vi "Parse State Queue++.vi"(0 "State Queue":string, 1 "Name(\"\" to use uuid)":string, 2 "Response Arguments":string, 7 "Error In (no error)":errorcluster, 9 "Dequeue Timeout(0ms)":i32, 11 "Response Timeout(5000ms)":i32=5000, 12 "Allowed Messages(Empty for all)":string[](array[string])) -> (3 "Name Used":string, 4 "Remaining States":string, 6 "Current State":string, 8 "Arguments":string, 10 ">> Response Source Message >>":T1, 15 ">> Source CSM >>":string)   [LabVIEW 2020, in "Communicable State Machine.lvlib"]
doc: "Parses the CSM state queue and returns the current state that will execute next with the associated arguments.\n\n\n<b>Inputs:</b>\n - <b>State Queue</b>: The entire state queue is wired to this input. This should come from the main CSM shift register.\n - <b>Error In (no error)</b>: The error cluster from the CSM is wired to this input. If an error occures and appears on this input, the current state output returns the \"Error Handler\" state.\n - <b>Name(\"\" to use uuid)</b>: Module Name\n - If Input is \"\", an uuid will be used for module name. The module is marked as stand-alone mode and will not be included in module list.\n - Fi Input end with '#', the module will worked in worker mode. Modules with the same name will shared the same message queue. Any external message will be processed by one of the modules, depends on who is free.\n - Otherwise, the input string will be used as module name, which should be unique in system. CSM will go to \"Critical Error\" state if duplicated module name is used in system.\n - <b>Response Timeout(5000ms)</b>: The timeout of waiting for response of sync-call from outside.\n - <b>Dequeue Timeout(0ms)</b>: The timeout of checking CSM message queue.\n - <b>Response Arguments</b>: The response arguments from last state. It should come from the CSM shift register.\n\n<b>Outputs:</b>\n - <b>Remaining States</b>: Returns all the next states that should execute after the current state completes. These should be passed through the current state in the state machine. These can also be modified or augmented within the current state if necessary.\n - <b>Arguments</b>: Returns any argument(s) that may be used in the current state string. These arguments come after the \">>\" characters. <b>Note:</b> The arguments variable must not contain any unprintable characters like linefeed or carriage return.\n - <b>Current State</b>: The state to be processed\n - <b>Name Used</b>: The actual name assigned to this CSM module\n - <b>Argument - State</b>: If any core error occurs, this is the source state name\n - <b>From Who</b>: If <b>Current State</b> is called by ouside, this is the source CSM module name."
uses:
  Communicable State Machine.lvlib
  _CSM_Response Source Message.ctl
  _CSM_GlobalLog_MSG.ctl
  _CSM_GlobalLog_MSG_TYPE.ctl
  Priority Queue.lvclass/Priority Queue.ctl
  _CSM_MSG_TYPE.ctl
  _CSM Status Change Event Data.ctl
  _CSMObj-Message Check.vi
  _CSMObj-Enqueue Cross-Module Message.vi
  _CSMOFGV Get.vi
  GEvt-Generate with Rule Check.vi
  Cache-Broadcast Registry Search Result.vi
  CSM - Register Status Change.vi
  CSM - Unregister Status Change.vi
  Hex Str to U8 Data.vi
  CSM - Revert Arguments-Safe String.vi
  Add State(s) to Queue__JKI_lib_State_Machine.vi
  Build Internal State String.vi
  Concatenate State with Arguments.vi
  U8 Data to Hex Str.vi
  Dequeue Element.vi
  CSM - Make String Arguments Safe.vi
  Enqueue Element.vi
  Filter Check.vi
  Trim Both Whitespace.vi
  CSM - Keywords.vi
  global-GEvnt Filter Change Flag.vi
  FGV-GEvt Filter Obj.vi
  Group Check - CSM.vi
  Group Check - LogType.vi
  Group Check - State.vi
  CSM Check - LogType.vi
  CSM Check - State.vi
  CSM Check - StateType.vi
  Group Check - StateType.vi
  _CSMOFGV.vi
  CSM Not Allowed Message.vi
  global-CSMQ FGV Change Flag.vi
  global-Broadcast Cache Change Flag.vi
  Broadcast Item Key.vi
  FGV-BroadcastRegistry.vi
  Parse Register Message.vi
  Parse Unregister Message.vi
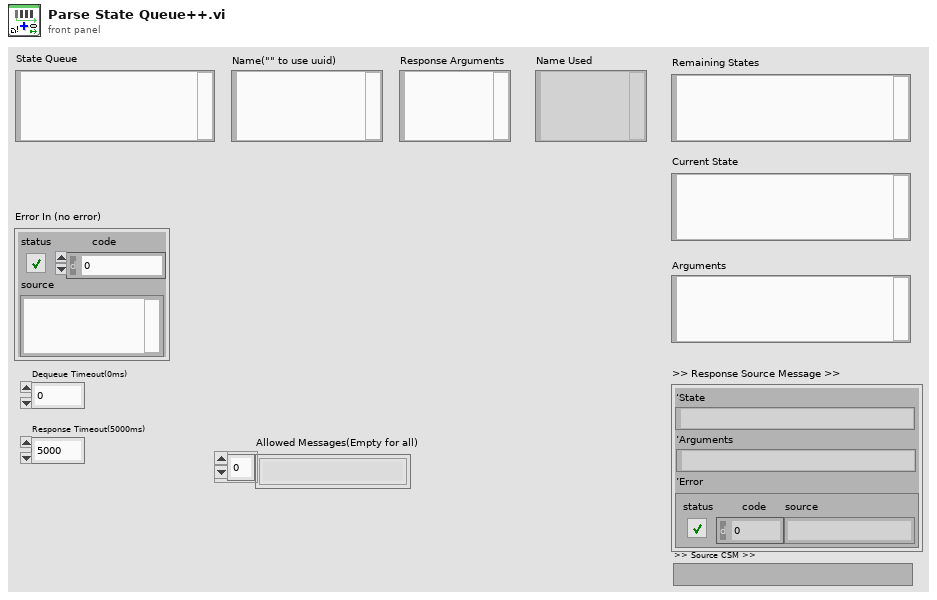
[diagram p1: front panel]
types:
  T1 = typedef "Communicable State Machine.lvlib/_CSM_Response Source Message.ctl" = cluster{"‘State":string, "’Arguments":string, "’Error":errorcluster}
  T2 = typedef "Communicable State Machine.lvlib/_CSM_GlobalLog_MSG.ctl" = cluster{"Name(\"\" to use uuid)":string, "Current State":string, "Arguments":string, "Source Message":T1, "Source Module":string, "Complete(T)/Start(F)":bool, "LogType":T3}
  T3 = typedef "Communicable State Machine.lvlib/_CSM_GlobalLog_MSG_TYPE.ctl" = enum16{"User Log", "State Change", "Status", "Interrupt", "Register", "Unregister", "Error Log", "Module Created", "Module Destroyed"}
  T4 = typedef "Communicable State Machine.lvlib/_CSMObj.ctl" = cluster{"Requested Name":string, "Module Name":string, "Mode":T5, "Queue":refnum<class "Priority Queue.lvclass">, "CSM-Data":refnum<data-value>, "User Event":refnum<user-event>, "Status Change Event":refnum<user-event>, "Allowed Messages":string[], "Mode-Data":refnum<data-value>, "Group Name":string, "Exit Event":refnum<user-event>}
  T5 = typedef "Communicable State Machine.lvlib/_CSM_MODE.ctl" = enum16{"Not Exist", "Stand Alone", "CSM", "Worker Agent", "Worker", "Chain", "Chain Node"}
  T6 = typedef "Communicable State Machine.lvlib/_CSM_MSG_TYPE.ctl" = enum16{"Sync Message(-@)", "Async Message(->)", "Async without Response(->|)", "Async Response", "Broadcast(-><all>)", "Broadcast(-><status>)", "Broadcast(-><interrupt>)", "Append to JKISM States", "Append to JKISM States(High Priority)"}
  T7 = typedef "Communicable State Machine.lvlib/_CSM Status Change Event Data.ctl" = cluster{"ModuleName":string, "Status":string, "Arguments":string}
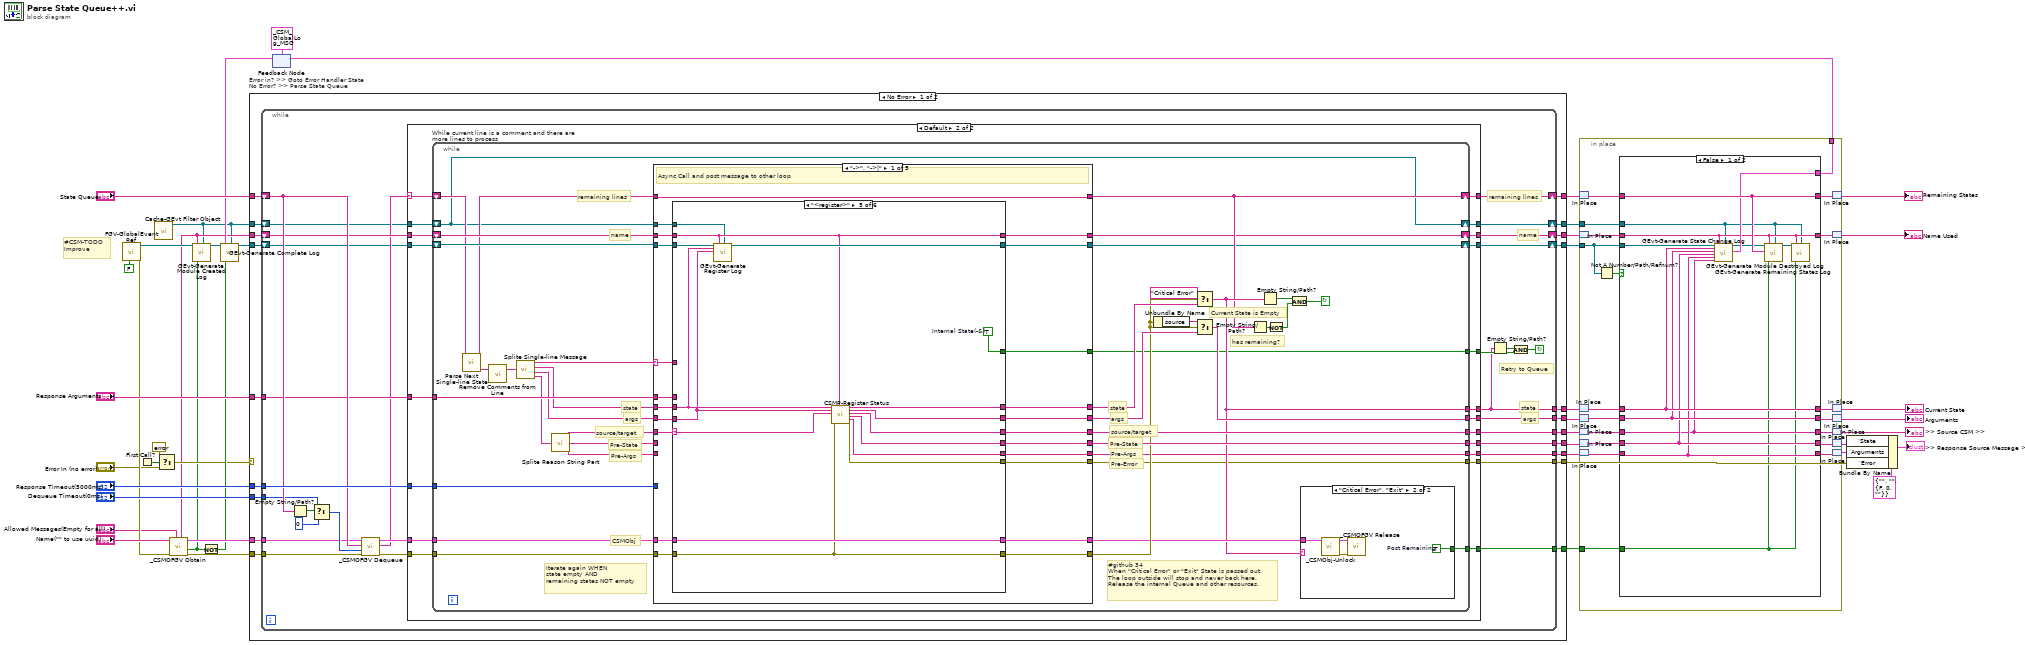
[diagram p0: block diagram]
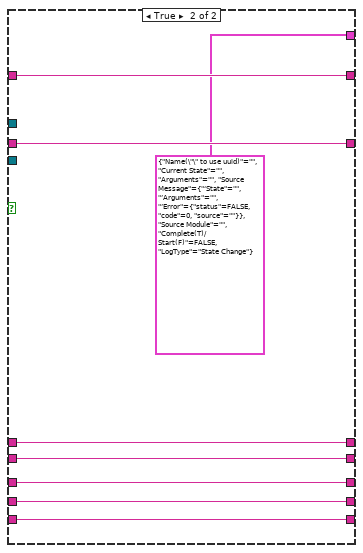
[diagram p2: hidden frame]
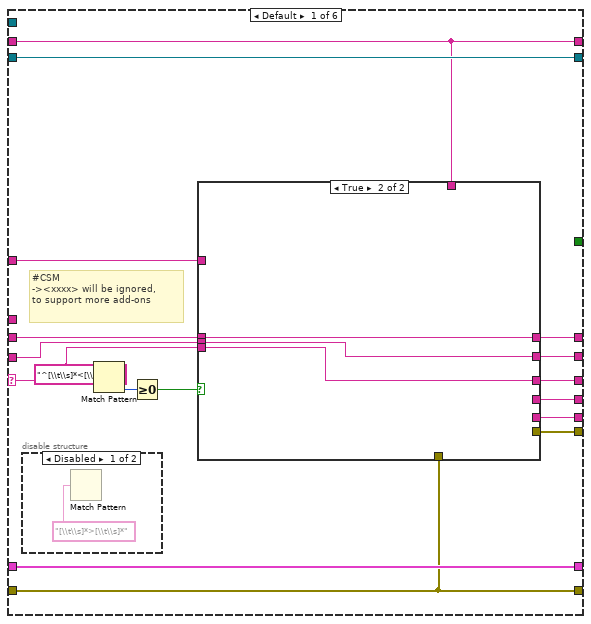
[diagram p5: hidden frame]
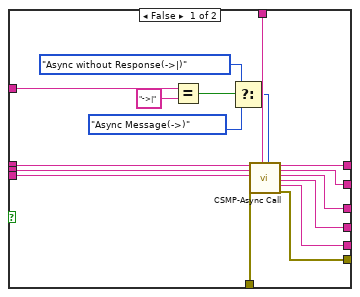
[diagram p7: hidden frame]
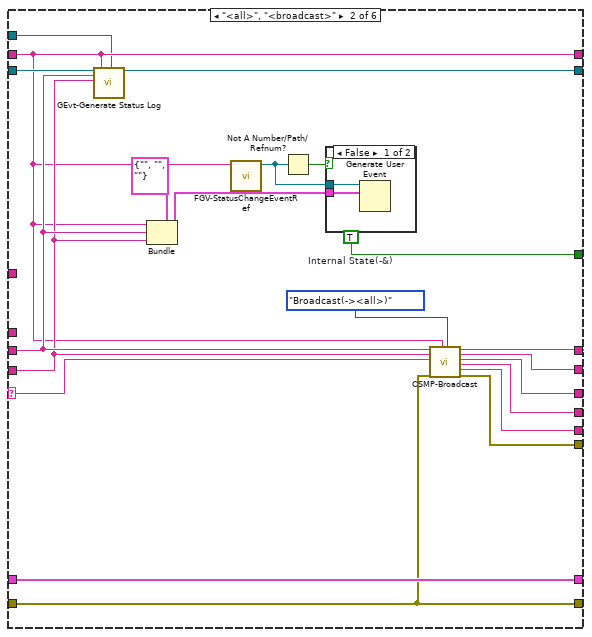
[diagram p8: hidden frame]
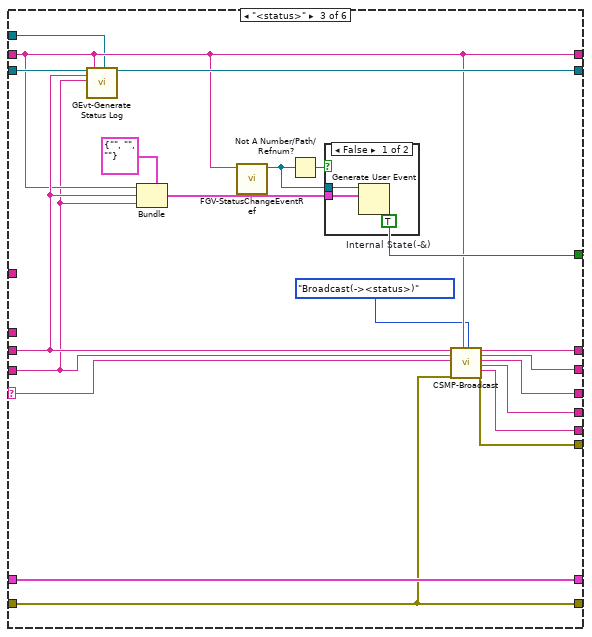
[diagram p10: hidden frame]
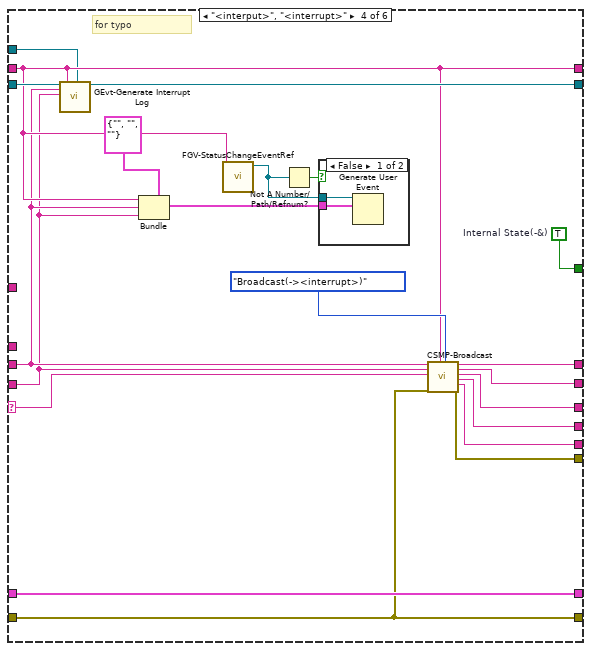
[diagram p12: hidden frame]
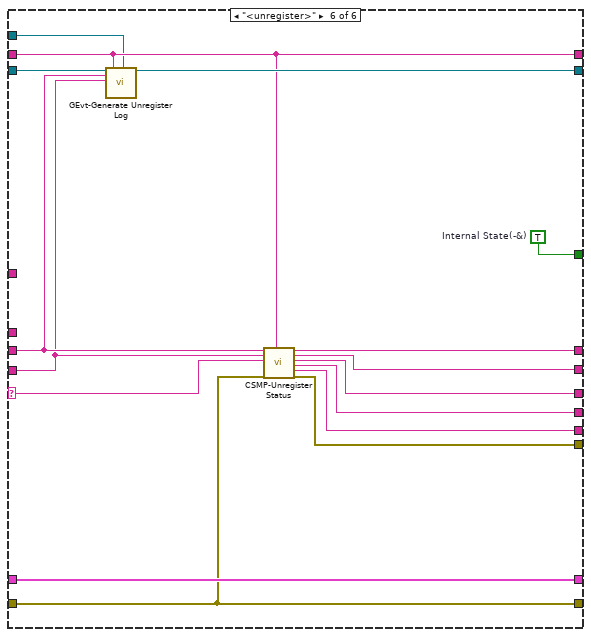
[diagram p14: hidden frame]
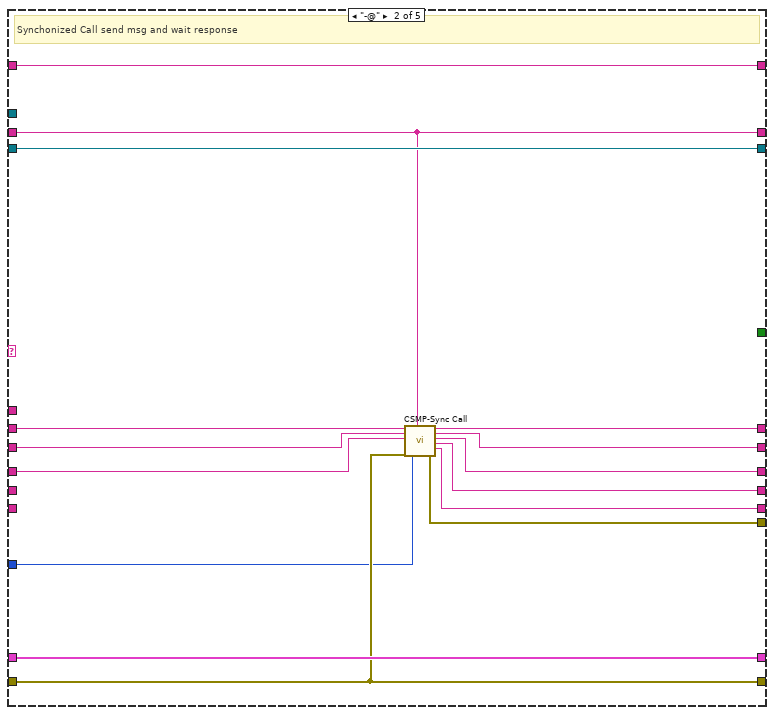
[diagram p15: hidden frame]
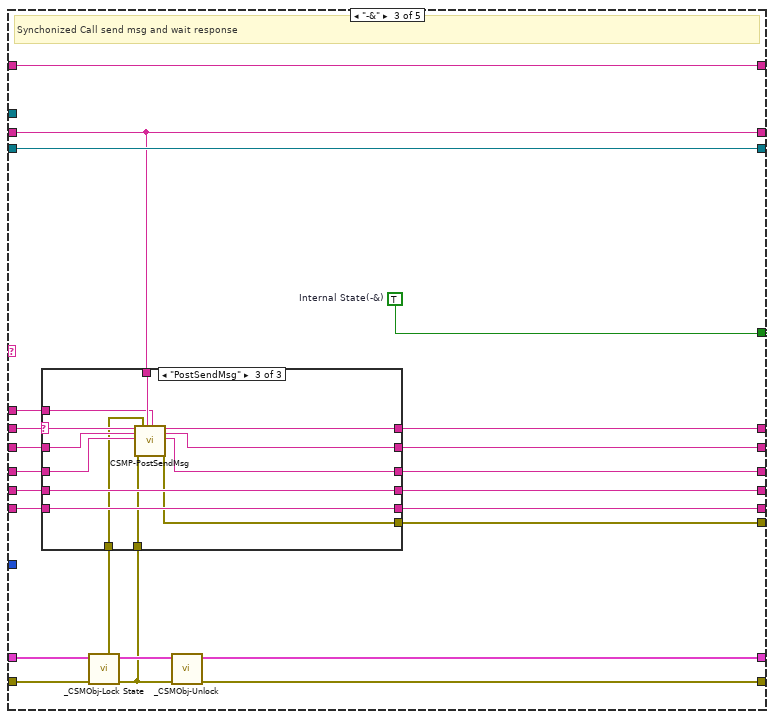
[diagram p16: hidden frame]
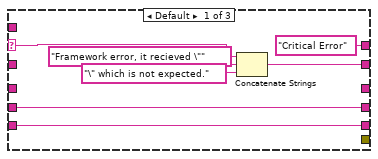
[diagram p17: hidden frame]
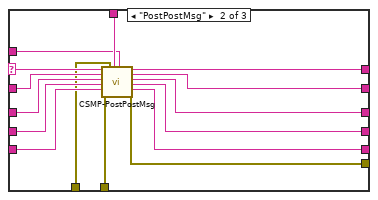
[diagram p18: hidden frame]
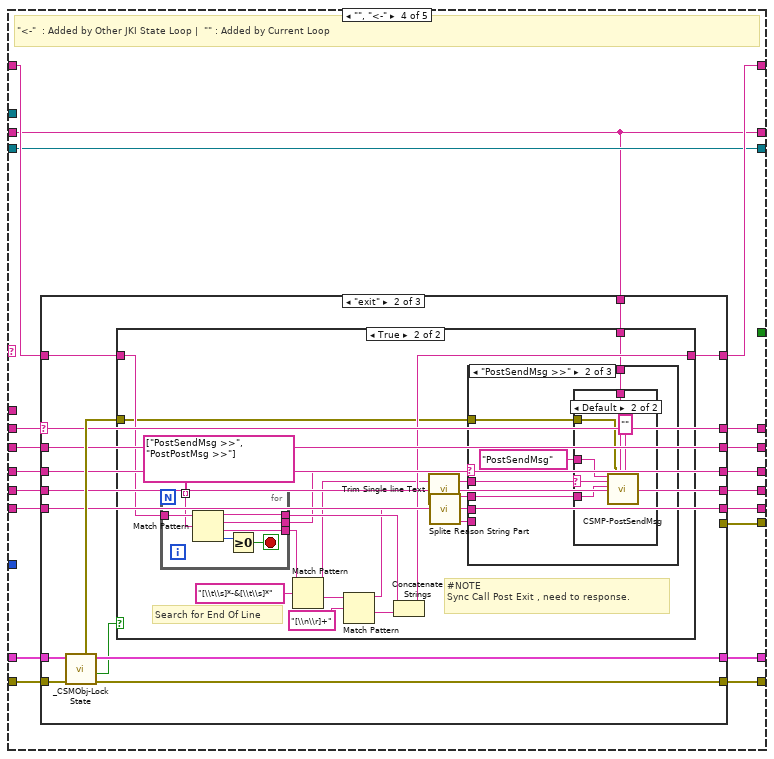
[diagram p19: hidden frame]
diagram:
  # "#CSM-TODO\nImprove"
  n1 = call "FGV-GlobalEventRef.vi"("Create(F)"=FALSE) -> ("error out"=w25:errorcluster, "CSM Global Log Event"=w6:refnum<user-event>)  [unwired: 9 in]
  n2 = First Call?() -> (First Call?: T/F=w10:bool)
  n3 = call "Cache-GEvt Filter Object.vi"() -> ("CSM:LogFilter.lvclass"=w1:refnum<class "LogFilter.lvclass">)  [unwired: 11 in]
  n4 = Select(t=errorcluster {"status"=FALSE, "code"=0, "source"=""}, s=w10, f="Error In (no error)") -> (s? t:f=w8:errorcluster)
  n5 = call "_CSMOFGV Obtain.vi"("Allowed Messages(Empty for all)"="Allowed Messages(Empty for all)", "Error in"=w25, "Name(\"\" to use uuid) in"="Name(\"\" to use uuid)") -> ("Error out"=w40:errorcluster, "Create(T)/Cached(F)"=w3:bool, "CSM-Obj"=w39:T4, "Name"=w4:string)  [unwired: 5 in]
  n6 = call "GEvt-Generate Module Created Log.vi"("CSM Global Log Event"=w6, "Name(\"\" to use uuid)"=w4, "Created?"=w3, "CSM:LogFilter.lvclass"=w1) -> ("CSM Global Log Event out"=w5:refnum<user-event>)  [unwired: 14 in, 1 out]
  n7 = Not(x=w3) -> (.not. x?=w11:bool)
  n8 = feedback #1(T2 {"Name(\"\" to use uuid)"="", "Current State"="", "Arguments"="", "Source Message"={"‘State"="", "’Arguments"="", "’Error"={"status"=FALSE, "code"=0, "source"=""}}, "Source Module"="", "Complete(T)/Start(F)"=FALSE, "LogType"=enum."State Change"} ("event data")) -> (w16:T2)
  n9 = call "GEvt-Generate Complete Log.vi"("CSM Global Log Event"=w5, "event data"=w16, "Enable?"=w11, "CSM:LogFilter.lvclass"=w1) -> ("CSM Global Log Event out"=w15:refnum<user-event>)  [unwired: 15 in]
  n10 = case "Error in? >> Goto Error Handler State\nNo Error? >> Parse State Queue" shown="No Error" w8 {
    selector: w8 -> [_ w508]
    tunnel: [w62 w515] -> w29
    tunnel: [w64 "Error Handler"] -> w38
    tunnel: [w63 w511] -> w37
    tunnel: "State Queue" -> [w59 w515]
    tunnel: "Response Timeout(5000ms)" -> [w61 _]
    tunnel: w39 -> [w54 w510]
    tunnel: [w60 _] -> w35
    tunnel: "Dequeue Timeout(0ms)" -> [w58 _]
    tunnel: [w57 _] -> w36
    tunnel: "Response Arguments" -> [w56 _]
    tunnel: w40 -> [w55 w509]
    tunnel: w4 -> [w53 w513]
    tunnel: [w52 _] -> w30
    tunnel: w15 -> [w51 w512]
    tunnel: [w50 w513] -> w24
    tunnel: [w49 w512] -> w23
    tunnel: [w48 _] -> w19
    tunnel: [w47 _] -> w13
    tunnel: w1 -> [w46 w507]
    tunnel: [w45 w507] -> w2
    frame No Error {
      n11 = while {
        tunnel: [w93] -> w63
        tunnel: w61 -> [w91]
        tunnel: [w90] -> w60
        tunnel: w58 -> [w86]
        tunnel: w55 -> [w81]
        tunnel: w54 -> [w80]
        shift-right: [w92] -> w62
        shift-left: w59 -> [w87]
        tunnel: w56 -> [w82]
        tunnel: [w74] -> w64
        tunnel: [w83] -> w57
        tunnel: [w72] -> w52
        shift-right: [w70] -> w50
        shift-left: w53 -> [w79]
        shift-right: [w69] -> w49
        shift-left: w51 -> [w71]
        tunnel: [w68] -> w48
        tunnel: [w67] -> w47
        shift-right: [w65] -> w45
        shift-left: w46 -> [w66]
        stop <- w76 continue-if-true
        # "args"
        # "state"
        # "name"
        # "remaining lines"
        # "Retry to Queue"
        n12 = Empty String/Path?(string/path=w87) -> (empty?=w88:bool)
        n13 = Select(t=w86, s=w88, f=0) -> (s? t:f=w84:i32)
        n14 = call "_CSMOFGV Dequeue.vi"("Error in"=w81, "Dequeue Timeout(0ms)"=w84, "State(s) in (\"\")"=w87, "CSMQ in"=w80) -> ("Error out"=w77:errorcluster, "States Out"=w78:string, "CSMQ out"=w89:T4)  [unwired: 5 in]
        n15 = case shown="Default" w78 {
          selector: w78 -> [_ w110]
          tunnel: [_ w116] -> w74
          tunnel: [_ w115] -> w93
          tunnel: [_ w114] -> w92
          tunnel: w91 -> [_ w113]
          tunnel: [_ w112] -> w90
          tunnel: w79 -> [w96 w111]
          tunnel: w89 -> [_ w109]
          tunnel: w77 -> [_ w108]
          tunnel: [_ w107] -> w83
          tunnel: w82 -> [_ w106]
          tunnel: [_ w105] -> w75
          tunnel: [_ w104] -> w72
          tunnel: w71 -> [w95 w103]
          tunnel: [w96 w102] -> w70
          tunnel: [w95 w101] -> w69
          tunnel: [_ w100] -> w68
          tunnel: [_ w99] -> w67
          tunnel: w66 -> [w94 w98]
          tunnel: [w94 w97] -> w65
          frame "" {
            # "Dispatch Mode\n1. Error will Occurred\n2. Add Macro: Exit\n3. The Queue will regenerated\n4. But it will go Through Macro: Exit\n5. After Exit(queue released), then another Worker will be triggered."
            # "Do Nothing if Empty String"
            # "<< Wiring into the Case Selector is much more performant than using \"Empty String/Path?\" primitive"
          }
          frame Default {
            n16 = while "While current line is a comment and there are more lines to process" {
              tunnel: [w141] -> w116
              tunnel: [w144] -> w115
              shift-right: [w135] -> w114
              shift-left: w110 -> [w127]
              tunnel: w113 -> [w152]
              tunnel: [w143] -> w112
              tunnel: w109 -> [w151]
              tunnel: w108 -> [w148]
              tunnel: [w150] -> w107
              tunnel: w106 -> [w149]
              tunnel: [w138] -> w105
              tunnel: [w136] -> w104
              shift-right: [w119] -> w102
              shift-left: w111 -> [w134]
              shift-right: [w118] -> w101
              shift-left: w103 -> [w133]
              tunnel: [w132] -> w100
              tunnel: [w120] -> w99
              shift-right: [w117] -> w97
              shift-left: w98 -> [w117]
              stop <- w137 continue-if-true
              # "source/target"
              # "Pre-Error"
              # "args"
              # "state"
              # "Pre-Args"
              # "Pre-State"
              # "source/target"
              # "Pre-Args"
              # "Pre-State"
              # "CSMObj"
              # "#github 34\nWhen \"Critical Error\" or \"Exit\" State is passed out,\nThe loop outside will stop and never back here.\nRelease the internal Queue and other resources."
              # "name"
              # "remaining lines"
              # "Iterate again WHEN\nstate empty AND\nremaining states NOT empty"
              # "args"
              # "state"
              # "Current State is Empty"
              # "has remaining?"
              n17 = call "Parse Next Single-line State.vi"("States Queue"=w127) -> ("Next Single-line State"=w125:string, "Remaining States Queue"=w126:string)  [unwired: 9 in]
              n18 = call "Remove Comments from Line.vi"("single-line text"=w125) -> ("single-line text without comments"=w131:string)  [unwired: 2 in]
              n19 = call "Splite Single-line Message.vi"("single-line text"=w131) -> ("operator"=w128:string, "state"=w129:string, "args"=w130:string, "source/target"=w124:string)  [unwired: 6 in]
              n20 = call "Splite Reason String Part.vi"("Single-line -& Reason"=w124) -> ("CSM Name"=w123:string, "`State"=w122:string, "`Arguments"=w121:string)  [unwired: 12 in]
              n21 = case shown="\"->\", \"->|\"" w128 {
                selector: w128 -> [w170 _ _ _ _]
                tunnel: w129 -> [w178 w331 w353 w405 w506]
                tunnel: w130 -> [w177 w330 w356 w403 w505]
                tunnel: [w181 w328 w358 w402 w506] -> w147
                tunnel: [w180 w327 w357 w401 w505] -> w146
                tunnel: w134 -> [w176 w332 w346 w404 w499]
                tunnel: w123 -> [w179 w329 w345 w399 w502]
                tunnel: w152 -> [_ w321 _ _ _]
                tunnel: w151 -> [w168 w335 w340 w412 w503]
                tunnel: w126 -> [w171 w334 w349 w408 w501]
                tunnel: [w175 w325 w352 w398 _] -> w150
                tunnel: w149 -> [w173 _ w355 _ _]
                tunnel: w148 -> [w174 w322 w339 w411 w504]
                tunnel: [w161 w322 w354 w410 w504] -> w145
                tunnel: [w163 w326 w342 w400 w502] -> w143
                tunnel: [w169 w335 w351 w409 w503] -> w142
                tunnel: [w172 _ w350 _ _] -> w138
                tunnel: [w171 w334 w349 w407 w501] -> w135
                tunnel: w133 -> [w167 w333 w348 w406 w500]
                tunnel: [w166 w333 w348 w406 w500] -> w118
                tunnel: [w164 w324 w347 w396 _] -> w132
                tunnel: [w165 w332 w346 w404 w499] -> w119
                tunnel: w122 -> [_ _ w344 w397 _]
                tunnel: w121 -> [_ _ w343 w395 _]
                tunnel: [w162 w323 w341 w394 _] -> w120
                tunnel: w117 -> [w160 _ _ _ _]
                frame "->", "->|" {
                  # "Async Call and post message to other loop"
                  n22 = case shown="\"<register>\"" w179 {
                    selector: w179 -> [w184 w228 w249 w273 w296 w312]
                    tunnel: [w192 w221 w252 w272 w295 w311] -> w181
                    tunnel: [w191 w222 w248 w271 w294 w310] -> w180
                    tunnel: w178 -> [w198 w232 w253 w275 w298 w315]
                    tunnel: w177 -> [w193 w231 w250 w274 w297 w313]
                    tunnel: w176 -> [w194 w230 w251 w277 w300 w314]
                    tunnel: [w190 w224 w246 w269 w292 w308] -> w175
                    tunnel: w174 -> [w186 w227 w255 w276 w299 w316]
                    tunnel: w173 -> [_ _ _ _ _ _]
                    tunnel: [_ w240 w263 w286 w304 w320] -> w172
                    tunnel: w170 -> [w197 _ _ _ _ _]
                    tunnel: [w196 w236 w262 w282 w303 w319] -> w169
                    tunnel: w168 -> [w196 w236 w262 w282 w303 w319]
                    tunnel: [w195 w234 w256 w279 w301 w317] -> w166
                    tunnel: w167 -> [w195 w233 w257 w280 w302 w318]
                    tunnel: [w194 w230 w251 w277 w300 w314] -> w165
                    tunnel: [w189 w225 w245 w268 w291 w307] -> w164
                    tunnel: [w188 w223 w247 w270 w293 w309] -> w163
                    tunnel: [w187 w226 w254 w267 w290 w306] -> w162
                    tunnel: [w186 w227 w255 w276 w299 w316] -> w161
                    tunnel: w160 -> [_ w220 w243 w266 w289 w305]
                    frame Default {
                      # "#CSM\n-><xxxx> will be ignored,\nto support more add-ons"
                      n23 = disable-structure shown="Disabled" {
                        frame Disabled {
                          n24 = Match Pattern(regular expression="[\\t\\s]*>[\\t\\s]*") -> ()  [unwired: 2 in, 4 out]
                        }
                        frame Enabled {
                        }
                      }
                      n25 = Match Pattern(string=w184, regular expression="^[\\t\\s]*<[\\t\\s]*") -> (offset past match=w183:i32)  [unwired: 1 in, 3 out]
                      n26 = Greater Or Equal To 0?(x=w183) -> (x >= 0?=w182:bool)
                      n27 = case shown="True" w182 {
                        tunnel: w198 -> [w216 w219]
                        tunnel: w197 -> [w215 _]
                        tunnel: w194 -> [w214 _]
                        tunnel: w193 -> [w213 w218]
                        tunnel: [w208 w219] -> w192
                        tunnel: [w207 w218] -> w191
                        tunnel: [w206 _] -> w190
                        tunnel: [w205 _] -> w189
                        tunnel: [w204 w217] -> w188
                        tunnel: [w203 _] -> w187
                        tunnel: w186 -> [w201 _]
                        tunnel: w184 -> [w200 w217]
                        frame False {
                          n28 = Equal?(x=w215, y="->|") -> (x = y?=w211:bool)
                          n29 = Select(t=_CSM_MSG_TYPE."Async without Response(->|)" ("Msg Type"), s=w211, f=_CSM_MSG_TYPE."Async Message(->)" ("Msg Type")) -> (s? t:f=w202:T6)
                          n30 = call "CSMP-Async Call.vi"("state"=w216, "args"=w213, "source/target"=w200, "Error in"=w201, "Module Name"=w214, "Msg Type"=w202) -> ("state out"=w208:string, "args out"=w207:string, "source/target out"=w204:string, "Pre-State out"=w206:string, "Pre-Args out"=w205:string, "error"=w203:errorcluster)  [unwired: 8 in]
                        }
                        frame True {
                        }
                      }
                    }
                    frame "<all>", "<broadcast>" {
                      w240 = TRUE  # Internal State(-&)
                      n31 = call "GEvt-Generate Status Log.vi"("CSM Global Log Event"=w233, "Current State"=w232, "Arguments"=w231, "Name(\"\" to use uuid)"=w230, "CSM:LogFilter.lvclass"=w220) -> ("CSM Global Log Event out"=w234:refnum<user-event>)  [unwired: 13 in, 1 out]
                      n32 = Bundle(cluster=T7 {"ModuleName"="", "Status"="", "Arguments"=""} ("event data"), "ModuleName"=w230, "Status"=w232, "Arguments"=w231) -> (w237:T7)
                      n33 = call "FGV-StatusChangeEventRef.vi"("Name(\"\" to use uuid) in"=w230) -> ("Status Change Event"=w235:refnum<user-event>)  [unwired: 9 in, 1 out]
                      n34 = Not A Number/Path/Refnum?(number/path/refnum=w235) -> (NaN/Path/Refnum?=w239:bool)
                      n35 = case shown="False" w239 {
                        tunnel: w235 -> [w242 _]
                        tunnel: w237 -> [w241 _]
                        frame False {
                          n36 = Generate User Event(user event=w242, event data cluster=w241) -> ()  [unwired: 2 in, 2 out]
                        }
                        frame True {
                        }
                      }
                      n37 = call "CSMP-Broadcast.vi"("state"=w232, "args"=w231, "source/target"=w228, "Error in"=w227, "Module Name"=w230, "Msg Type"=_CSM_MSG_TYPE."Broadcast(-><all>)") -> ("state out"=w221:string, "args out"=w222:string, "source/target out"=w223:string, "Pre-State out"=w224:string, "Pre-Args out"=w225:string, "error"=w226:errorcluster)  [unwired: 8 in]
                    }
                    frame "<status>" {
                      w263 = TRUE  # Internal State(-&)
                      n38 = call "GEvt-Generate Status Log.vi"("CSM Global Log Event"=w257, "Current State"=w253, "Arguments"=w250, "Name(\"\" to use uuid)"=w251, "CSM:LogFilter.lvclass"=w243) -> ("CSM Global Log Event out"=w256:refnum<user-event>)  [unwired: 13 in, 1 out]
                      n39 = Bundle(cluster=T7 {"ModuleName"="", "Status"="", "Arguments"=""} ("event data"), "ModuleName"=w251, "Status"=w253, "Arguments"=w250) -> (w259:T7)
                      n40 = call "FGV-StatusChangeEventRef.vi"("Name(\"\" to use uuid) in"=w251) -> ("Status Change Event"=w258:refnum<user-event>)  [unwired: 9 in, 1 out]
                      n41 = Not A Number/Path/Refnum?(number/path/refnum=w258) -> (NaN/Path/Refnum?=w261:bool)
                      n42 = case shown="False" w261 {
                        tunnel: w258 -> [w265 _]
                        tunnel: w259 -> [w264 _]
                        frame False {
                          n43 = Generate User Event(user event=w265, event data cluster=w264) -> ()  [unwired: 2 in, 2 out]
                        }
                        frame True {
                        }
                      }
                      n44 = call "CSMP-Broadcast.vi"("state"=w253, "args"=w250, "source/target"=w249, "Error in"=w255, "Module Name"=w251, "Msg Type"=_CSM_MSG_TYPE."Broadcast(-><status>)") -> ("state out"=w252:string, "args out"=w248:string, "source/target out"=w247:string, "Pre-State out"=w246:string, "Pre-Args out"=w245:string, "error"=w254:errorcluster)  [unwired: 8 in]
                    }
                    frame "<interput>", "<interrupt>" {
                      w286 = TRUE  # Internal State(-&)
                      # "for typo"
                      n45 = call "GEvt-Generate Interrupt Log.vi"("CSM Global Log Event"=w280, "Current State"=w275, "Arguments"=w274, "Name(\"\" to use uuid)"=w277, "CSM:LogFilter.lvclass"=w266) -> ("CSM Global Log Event out"=w279:refnum<user-event>)  [unwired: 13 in, 1 out]
                      n46 = Bundle(cluster=T7 {"ModuleName"="", "Status"="", "Arguments"=""} ("event data"), "ModuleName"=w277, "Status"=w275, "Arguments"=w274) -> (w283:T7)
                      n47 = call "FGV-StatusChangeEventRef.vi"("Name(\"\" to use uuid) in"=w277) -> ("Status Change Event"=w281:refnum<user-event>)  [unwired: 9 in, 1 out]
                      n48 = Not A Number/Path/Refnum?(number/path/refnum=w281) -> (NaN/Path/Refnum?=w285:bool)
                      n49 = case shown="False" w285 {
                        tunnel: w281 -> [w288 _]
                        tunnel: w283 -> [w287 _]
                        frame False {
                          n50 = Generate User Event(user event=w288, event data cluster=w287) -> ()  [unwired: 2 in, 2 out]
                        }
                        frame True {
                        }
                      }
                      n51 = call "CSMP-Broadcast.vi"("state"=w275, "args"=w274, "source/target"=w273, "Error in"=w276, "Module Name"=w277, "Msg Type"=_CSM_MSG_TYPE."Broadcast(-><interrupt>)") -> ("state out"=w272:string, "args out"=w271:string, "source/target out"=w270:string, "Pre-State out"=w269:string, "Pre-Args out"=w268:string, "error"=w267:errorcluster)  [unwired: 8 in]
                    }
                    frame "<register>" {
                      w304 = TRUE  # Internal State(-&)
                      n52 = call "GEvt-Generate Register Log.vi"("CSM Global Log Event"=w302, "Current State"=w298, "Arguments"=w297, "Name(\"\" to use uuid)"=w300, "CSM:LogFilter.lvclass"=w289) -> ("CSM Global Log Event out"=w301:refnum<user-event>)  [unwired: 13 in, 1 out]
                      n53 = call "CSMP-Register Status.vi"("state"=w298, "args"=w297, "source/target"=w296, "Error in"=w299, "Module Name"=w300) -> ("state out"=w295:string, "args out"=w294:string, "source/target out"=w293:string, "Pre-State out"=w292:string, "Pre-Args out"=w291:string, "error"=w290:errorcluster)  [unwired: 9 in]
                    }
                    frame "<unregister>" {
                      w320 = TRUE  # Internal State(-&)
                      n54 = call "GEvt-Generate Unregister Log.vi"("CSM Global Log Event"=w318, "Current State"=w315, "Arguments"=w313, "Name(\"\" to use uuid)"=w314, "CSM:LogFilter.lvclass"=w305) -> ("CSM Global Log Event out"=w317:refnum<user-event>)  [unwired: 13 in, 1 out]
                      n55 = call "CSMP-Unregister Status.vi"("state"=w315, "args"=w313, "source/target"=w312, "Error in"=w316, "Module Name"=w314) -> ("state out"=w311:string, "args out"=w310:string, "source/target out"=w309:string, "Pre-State out"=w308:string, "Pre-Args out"=w307:string, "error"=w306:errorcluster)  [unwired: 9 in]
                    }
                  }
                }
                frame "-@" {
                  # "Synchonized Call send msg and wait response"
                  n56 = call "CSMP-Sync Call.vi"("state"=w331, "args"=w330, "source/target"=w329, "Error in"=w322, "Response Timeout(5000ms)"=w321, "Module Name"=w332) -> ("state out"=w328:string, "args out"=w327:string, "source/target out"=w326:string, "Pre-State out"=w325:string, "Pre-Args out"=w324:string, "error"=w323:errorcluster)  [unwired: 8 in]
                }
                frame "-&" {
                  w350 = TRUE  # Internal State(-&)
                  # "Synchonized Call send msg and wait response"
                  n57 = call "_CSMObj-Lock State.vi"("Error in"=w339, "CSMQ in"=w340) -> ("Error out"=w337:errorcluster, "CSMQ out"=w338:T4, "error"=w336:errorcluster)  [unwired: 5 in, 1 out]
                  n58 = case shown="\"PostSendMsg\"" w353 {
                    selector: w353 -> [w361 w376 w389]
                    tunnel: ["Critical Error" ("before match") w367 w388] -> w358
                    tunnel: [w363 w368 w385] -> w357
                    tunnel: w345 -> [_ w374 w386]
                    tunnel: w356 -> [_ w375 w387]
                    tunnel: w355 -> [_ w377 w390]
                    tunnel: w337 -> [_ w380 w383]
                    tunnel: w346 -> [_ w378 w391]
                    tunnel: [w360 w370 w393] -> w352
                    tunnel: w344 -> [w360 w373 w393]
                    tunnel: w343 -> [w359 w372 w392]
                    tunnel: [w359 w371 w392] -> w347
                    tunnel: [_ w379 w382] -> w341
                    tunnel: [_ w369 w384] -> w342
                    tunnel: w336 -> [_ w366 w381]
                    frame Default {
                      n59 = Concatenate Strings("Framework error, it recieved \"" ("before match"), w361, "\" which is not expected." ("before match")) -> (w363:string)
                    }
                    frame "PostPostMsg" {
                      n60 = call "CSMP-PostPostMsg.vi"("state"=w376, "args"=w375, "source/target"=w374, "Pre-State in"=w373, "Pre-Args in"=w372, "Error in"=w380, "session error"=w366, "Module Name"=w378, "Response Arguments"=w377) -> ("state out"=w367:string, "args out"=w368:string, "source/target out"=w369:string, "Pre-State out"=w370:string, "Pre-Args out"=w371:string, "error"=w379:errorcluster)  [unwired: 5 in]
                    }
                    frame "PostSendMsg" {
                      n61 = call "CSMP-PostSendMsg.vi"("state"=w389, "args"=w387, "source/target"=w386, "Error in"=w383, "session error"=w381, "Module Name"=w391, "Response Arguments"=w390) -> ("state out"=w388:string, "args out"=w385:string, "source/target out"=w384:string, "error"=w382:errorcluster)  [unwired: 9 in]
                    }
                  }
                  n62 = call "_CSMObj-Unlock.vi"("Error in"=w337, "CSMQ in"=w338) -> ("Error out"=w354:errorcluster, "CSMQ out"=w351:T4)  [unwired: 8 in]
                }
                frame "", "<-" {
                  # "\"<-\"  : Added by Other JKI State Loop |  \"\" : Added by Current Loop"
                  n63 = case shown="\"exit\"" w405 {
                    selector: w405 -> [w417 w425 w497]
                    tunnel: w408 -> [w418 w430 w498]
                    tunnel: w412 -> [w419 w434 w493]
                    tunnel: w411 -> [w420 w433 w492]
                    tunnel: [w420 w427 w492] -> w410
                    tunnel: [w419 w432 w493] -> w409
                    tunnel: [w418 w431 w498] -> w407
                    tunnel: w404 -> [_ w428 _]
                    tunnel: w403 -> [w416 w424 w496]
                    tunnel: [w417 w425 w497] -> w402
                    tunnel: [w416 w424 w496] -> w401
                    tunnel: [w415 w423 w495] -> w400
                    tunnel: w399 -> [w415 w423 w495]
                    tunnel: [w414 w422 w494] -> w398
                    tunnel: w397 -> [w414 w422 w494]
                    tunnel: [w413 w421 w489] -> w396
                    tunnel: w395 -> [w413 w421 w490]
                    tunnel: [_ _ w487] -> w394
                    frame Default {
                    }
                    frame "exit" {
                      n64 = call "_CSMObj-Lock State.vi"("Error in"=w433, "CSMQ in"=w434) -> ("Error out"=w427:errorcluster, "RemoteMessge?"=w429:bool, "CSMQ out"=w432:T4, "error"=w426:errorcluster)  [unwired: 5 in]
                      n65 = case shown="True" w429 {
                        tunnel: [w435 w450] -> w431
                        tunnel: w430 -> [w435 w445]
                        tunnel: w428 -> [_ w437]
                        tunnel: w426 -> [_ w436]
                        frame False {
                        }
                        frame True {
                          # "#NOTE\nSync Call Post Exit , need to response."
                          # "Search for End Of Line"
                          n66 = for {
                            tunnel: [w486] -> w452
                            tunnel: w445 -> [w484]
                            tunnel: [w485] -> w451
                            tunnel: string[] ["PostSendMsg >>", "PostPostMsg >>"] -> [w483] mode=indexing
                            tunnel: [w480] -> w443
                            stop <- w481 stop-if-true
                            n67 = Match Pattern(string=w484, regular expression=w483) -> (before substring=w485:string, match substring=w480:string, after substring=w486:string, offset past match=w482:i32)  [unwired: 1 in]
                            n68 = Greater Or Equal To 0?(x=w482) -> (x >= 0?=w481:bool)
                          }
                          n69 = Match Pattern(string=w452, regular expression="[\\t\\s]*-&[\\t\\s]*") -> (before substring=w446:string, after substring=w448:string)  [unwired: 1 in, 2 out]
                          n70 = Match Pattern(string=w448, regular expression="[\\n\\r]+") -> (before substring=w442:string, after substring=w447:string)  [unwired: 1 in, 2 out]
                          n71 = Concatenate Strings(w451, w447) -> (w450:string)
                          n72 = call "Trim Single line Text.vi"("single-line text"=w446) -> ("trimed text"=w438:string)  [unwired: 2 in]
                          n73 = call "Splite Reason String Part.vi"("Single-line -& Reason"=w442) -> ("CSM Name"=w441:string, "`State"=w440:string, "`Arguments"=w439:string)  [unwired: 12 in]
                          n74 = case shown="\"PostSendMsg >>\"" w443 {
                            tunnel: w438 -> [_ w458 w471]
                            tunnel: w441 -> [_ w457 w470]
                            tunnel: w440 -> [_ _ w468]
                            tunnel: w439 -> [_ _ w467]
                            tunnel: w437 -> [_ w455 w466]
                            tunnel: w436 -> [_ w454 w465]
                            frame Default {
                            }
                            frame "PostSendMsg >>" {
                              n75 = case shown="Default" w458 {
                                selector: w458 -> [_ w464]
                                tunnel: w457 -> [_ w463]
                                tunnel: "PostSendMsg" ("regular expression") -> [_ w461]
                                tunnel: w455 -> [_ w460]
                                tunnel: w454 -> [_ w459]
                                frame "" {
                                }
                                frame Default {
                                n76 = call "CSMP-PostSendMsg.vi"("state"=w461, "args"=w464, "source/target"=w463, "session error"=w459, "Module Name"=w460, "Response Arguments"="" ("Module Name")) -> ()  [unwired: 10 in, 4 out]
                                }
                              }
                            }
                            frame "PostPostMsg >>" {
                              n77 = case shown="Default" w471 {
                                selector: w471 -> [_ w477]
                                tunnel: w470 -> [_ w476]
                                tunnel: "PostPostMsg" ("regular expression") -> [_ w479]
                                tunnel: w468 -> [_ w475]
                                tunnel: w467 -> [_ w474]
                                tunnel: w466 -> [_ w473]
                                tunnel: w465 -> [_ w472]
                                frame "" {
                                }
                                frame Default {
                                n78 = call "CSMP-PostPostMsg.vi"("state"=w479, "args"=w477, "source/target"=w476, "Pre-State in"=w475, "Pre-Args in"=w474, "session error"=w472, "Module Name"=w473, "Response Arguments"="" ("Module Name")) -> ()  [unwired: 6 in, 6 out]
                                }
                              }
                            }
                          }
                        }
                      }
                    }
                    frame "async response" {
                      n79 = Match Pattern(string=w490, regular expression="[\\t\\s]*>>>[\\t\\s]*") -> (before substring=w489:string, after substring=w488:string)  [unwired: 1 in, 2 out]
                      n80 = call "CSM - Convert Argument to Error.vi"("Argument"=w488) -> ("error"=w487:errorcluster)  [unwired: 4 in]
                    }
                  }
                }
                frame Default {
                  # "Error, should not be here."
                }
              }
              n81 = Unbundle By Name(w145) -> ("source"=w140:string)
              n82 = Select(t="Critical Error", s=w145, f=w147) -> (s? t:f=w141:string)
              n83 = Select(t=w140, s=w145, f=w146) -> (s? t:f=w144:string)
              n84 = Empty String/Path?(string/path=w135) -> (empty?=w154:bool)
              n85 = Empty String/Path?(string/path=w141) -> (empty?=w155:bool)
              n86 = Not(x=w154) -> (.not. x?=w153:bool)
              n87 = And(x=w155, y=w153) -> (x .and. y?=w137:bool)
              n88 = case shown="\"Critical Error\", \"Exit\"" w141 {
                tunnel: w142 -> [_ w159]
                tunnel: [_ w157] -> w136
                frame "False", Default {
                }
                frame "Critical Error", "Exit" {
                  w157 = TRUE  # Post Remaining
                  n89 = call "_CSMObj-Unlock.vi"("CSMQ in"=w159) -> ("Error out"=w156:errorcluster, "CSMQ out"=w158:T4)  [unwired: 9 in]
                  n90 = call "_CSMOFGV Release.vi"("Error in"=w156, "CSMQ"=w158) -> ()  [unwired: 9 in, 1 out]
                }
              }
            }
          }
        }
        n91 = Empty String/Path?(string/path=w74) -> (empty?=w73:bool)
        n92 = And(x=w73, y=w75) -> (x .and. y?=w76:bool)
      }
    }
    frame Error {
      # "Goto Error Handler State >>"
      # "preserve remaining states >>"
      n93 = call "_CSMObj-Log Error if in a Remote Session.vi"("error"=w508, "Error in"=w509, "CSMQ in"=w510) -> ()  [unwired: 7 in, 2 out]
      n94 = call "CSM - Convert Error to Argument.vi"("error in (no error)"=w508) -> ("Arguments"=w511:string)  [unwired: 4 in]
    }
  }
  n95 = in-place {
    in-place-border: w30 -> [w523]
    in-place-border: w23 -> [w520]
    in-place-border: [w519] -> w22
    in-place-border: w2 -> [w516]
    n96 = in-place-match #2(w29) -> (w521:string)
    n97 = in-place-match #3(w24) -> (w529:string)
    n98 = in-place-match #4(w38) -> (w531:string)
    n99 = in-place-match #5(w37) -> (w532:string)
    n100 = in-place-match #6(w35) -> (w530:string)
    n101 = in-place-match #7(w36) -> (w533:string)
    n102 = in-place-match #8(w19) -> (w517:string)
    n103 = Not A Number/Path/Refnum?(number/path/refnum=w520) -> (NaN/Path/Refnum?=w534:bool)
    n104 = case shown="False" w534 {
      tunnel: w520 -> [w546 _]
      tunnel: w531 -> [w545 w555]
      tunnel: [w545 w555] -> w528
      tunnel: w532 -> [w544 w554]
      tunnel: [w544 w554] -> w527
      tunnel: [w543 w553] -> w526
      tunnel: w533 -> [w543 w553]
      tunnel: [w540 w552] -> w525
      tunnel: w530 -> [w540 w552]
      tunnel: w529 -> [w537 w551]
      tunnel: [w537 w551] -> w524
      tunnel: w523 -> [w536 _]
      tunnel: [w547 w550] -> w522
      tunnel: w521 -> [w547 w550]
      tunnel: [w541 T2 {"Name(\"\" to use uuid)"="", "Current State"="", "Arguments"="", "Source Message"={"‘State"="", "’Arguments"="", "’Error"={"status"=FALSE, "code"=0, "source"=""}}, "Source Module"="", "Complete(T)/Start(F)"=FALSE, "LogType"=enum."State Change"} ("event data")] -> w519
      tunnel: [w542 w549] -> w518
      tunnel: w517 -> [w542 w549]
      tunnel: w516 -> [w535 _]
      frame False {
        n105 = call "GEvt-Generate State Change Log.vi"("CSM Global Log Event"=w546, "Current State"=w545, "Arguments"=w544, "Source Message.*State"=w543, "Source Message.*Arguments"=w542, "Source Module"=w540, "Name(\"\" to use uuid)"=w537, "CSM:LogFilter.lvclass"=w535) -> ("CSM Global Log Event out"=w539:refnum<user-event>, "event data"=w541:T2)  [unwired: 10 in]
        n106 = call "GEvt-Generate Remaining States Log.vi"("CSM Global Log Event"=w539, "Remaining States"=w547, "Name(\"\" to use uuid)"=w537, "Enable?"=w536, "CSM:LogFilter.lvclass"=w535) -> ("CSM Global Log Event out"=w538:refnum<user-event>)  [unwired: 13 in, 1 out]
        n107 = call "GEvt-Generate Module Destroyed Log.vi"("CSM Global Log Event"=w538, "Name(\"\" to use uuid)"=w537, "Enable?"=w536, "CSM:LogFilter.lvclass"=w535) -> ()  [unwired: 14 in, 2 out]
      }
      frame True {
      }
    }
    n108 = in-place-match #2(w522) -> (→"Remaining States":string)
    n109 = in-place-match #3(w524) -> (→"Name Used":string)
    n110 = in-place-match #4(w528) -> (→"Current State":string)
    n111 = in-place-match #5(w527) -> (→"Arguments":string)
    n112 = in-place-match #6(w525) -> (→">> Source CSM >>":string)
    n113 = in-place-match #7(w526) -> (w21:string)
    n114 = in-place-match #8(w518) -> (w18:string)
  }
  n115 = feedback-in #1(w22) -> ()
  n116 = Bundle By Name(cluster=T1 {"‘State"="", "’Arguments"="", "’Error"={"status"=FALSE, "code"=0, "source"=""}} (">> Response Source Message >>"), "‘State"=w21, "’Arguments"=w18, "’Error"=w13) -> (→">> Response Source Message >>":T1)
